vi "Adjust_Arm_Direction.vi"(1 "Arm Direction":i16) -> (0 "Adjusted Direction":i16)   [LabVIEW 2012]
uses:
  climber_sensor_readings.ctl
panel:
  in  "Climber Inputs":T1
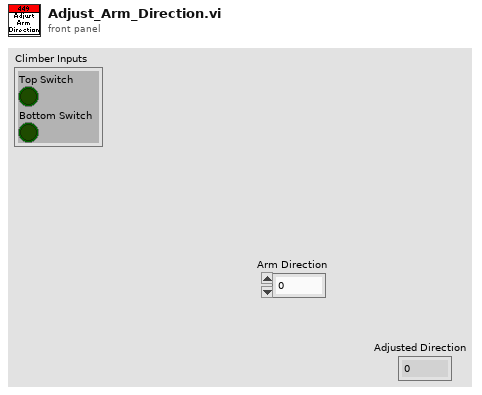
[diagram p1: front panel]
types:
  T1 = typedef "climber_sensor_readings.ctl" = cluster{"Top Switch":bool, "Bottom Switch":bool}
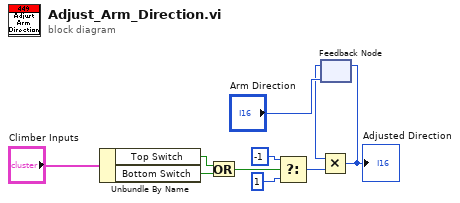
[diagram p0: block diagram]
diagram:
  n1 = Unbundle By Name("Climber Inputs") -> ("Top Switch"=w2:bool, "Bottom Switch"=w1:bool)
  n2 = Or(x=w2, y=w1) -> (x .or. y?=w4:bool)
  n3 = Select(t=i16 -1, s=w4, f=i16 1) -> (s? t:f=w8:i16)
  n4 = feedback #1("Arm Direction") -> (w5:i16)
  n5 = Multiply(x=w5, y=w8) -> (x*y=w6:i16)
  "Adjusted Direction" <- w6
  n6 = feedback-in #1(w6) -> ()
